vi "close.vi"(8 "error in (no error)":errorcluster, 11 "DMC1000B in":refnum<class "DMC1000B.lvclass">) -> (0 "error out":errorcluster, 3 "DMC1000B out":refnum<class "DMC1000B.lvclass">)   [LabVIEW 2019, in "DMC1000B.lvclass"]
uses:
  DMC1000B.lvclass
  LLB/DMC1000B/Dmc1000/Dmc1000.lvlib
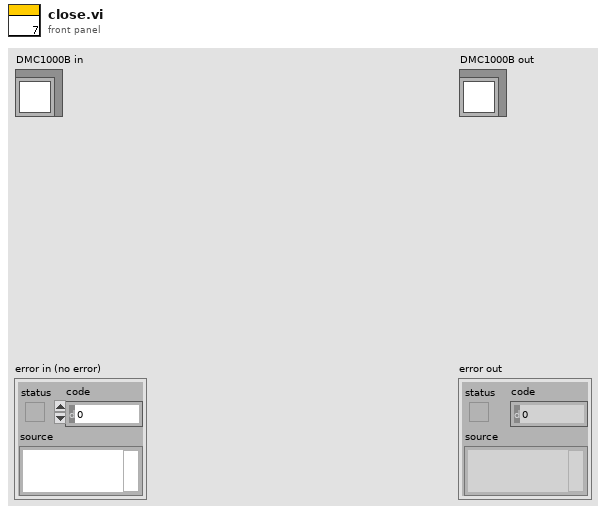
[diagram p1: front panel]
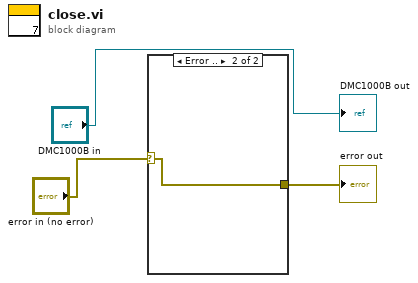
[diagram p0: block diagram]
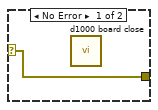
[diagram p2: hidden frame]
diagram:
  n1 = case shown="Error .." "error in (no error)" {
    selector: "error in (no error)" -> [w4 w5]
    tunnel: [w4 w5] -> w1
    frame No Error {
      n2 = call "d1000 board close.vi"() -> ()  [unwired: 11 in, 1 out]
    }
    frame Error {
    }
  }
  "error out" <- w1
  "DMC1000B out" <- "DMC1000B in"
